vi "Get Rx Monitor Queue Status Section and Channels.vi"(8 "error in":errorcluster, 11 "custom device ref in":T1 format="%.0x") -> (0 "error out":errorcluster, 1 "Rx monitor section channel refs":T1[](array[typedef]) format="%.0x", 2 "Rx monitor section ref out":T1 format="%.0x", 3 "custom device ref out":T1 format="%.0x", 4 "found?":bool)   [LabVIEW 2020, in "AIM ARINC 664 Scripting.lvlib"]
uses:
  AIM ARINC 664 Scripting.lvlib
  <vilib>/NI VeriStand/Custom Device API/Custom Device Item Ref.ctl
  Constants.vi
  <vilib>/NI VeriStand/Custom Device API/Custom Device API.lvlib
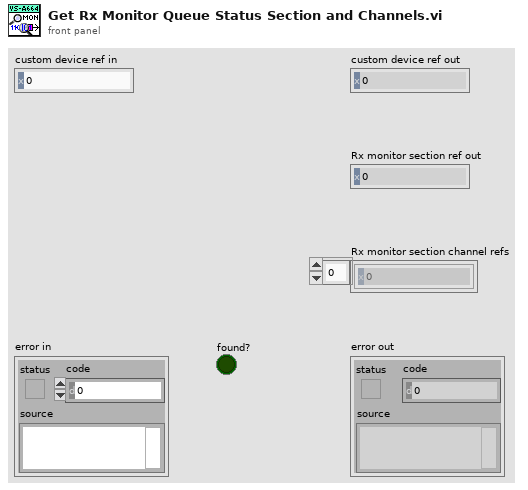
[diagram p1: front panel]
types:
  T1 = typedef "Custom Device API.lvlib/Custom Device Item Ref.ctl" = u64
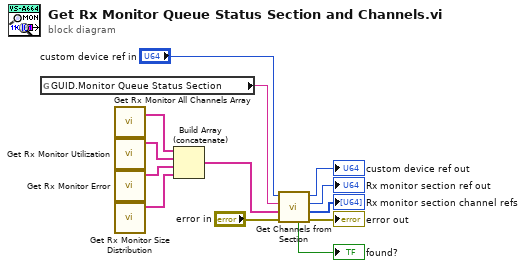
[diagram p0: block diagram]
diagram:
  n1 = global read "Constants.vi" "GUID.Monitor Queue Status Section"() -> (w9:string)
  n2 = call "Get Rx Monitor All Channels Array.vi"() -> ("channel array"=w13:string[])  [unwired: 3 in]
  n3 = call "Get Rx Monitor Utilization.vi"() -> ("channel array"=w12:string[])  [unwired: 11 in]
  n4 = call "Get Rx Monitor Error.vi"() -> ("channel array"=w11:string[])  [unwired: 11 in]
  n5 = call "Get Rx Monitor Size Distribution.vi"() -> ("channel array"=w10:string[])  [unwired: 11 in]
  n6 = Build Array (concatenate)(w13, w12, w11, w10) -> (w8:string[])
  n7 = call "Get Channels from Section.vi"("error in"="error in", "channel array names"=w8, "GUID section"=w9, "custom device ref in"="custom device ref in") -> ("error out"=→"error out":errorcluster, "channel array refs out"=→"Rx monitor section channel refs":T1[], "section ref out"=→"Rx monitor section ref out":T1, "custom device ref out"=→"custom device ref out":T1, "all channels found?"=→"found?":bool)  [unwired: 2 in, 1 out]
